vi "Set Control Size.vi"(7 "CtrlRef":refnum<vi>, 9 "Size":cluster{"Width":u32, "Height":u32}, 11 "error in (no error)":errorcluster) -> (15 "error out":errorcluster)   [LabVIEW 2011]
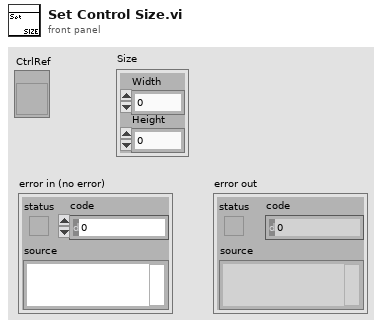
[diagram p1: front panel]
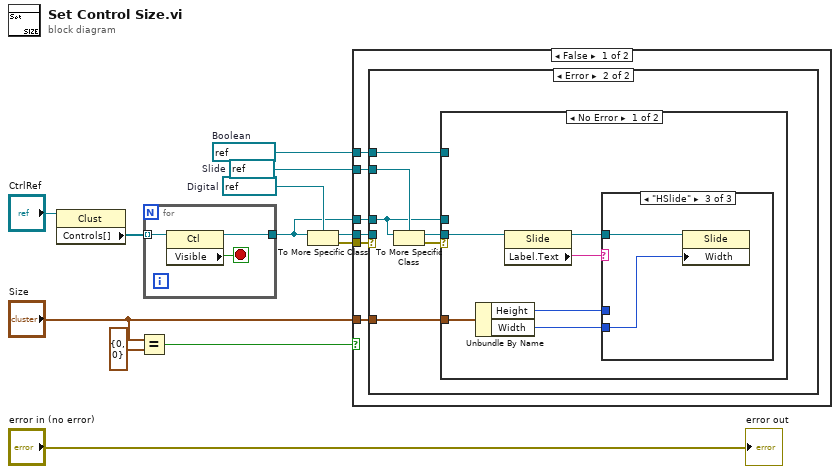
[diagram p0: block diagram]
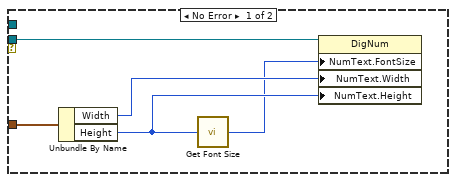
[diagram p2: hidden frame]
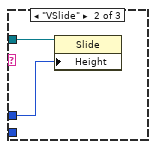
[diagram p4: hidden frame]
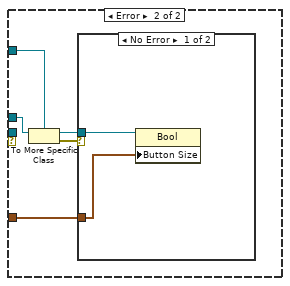
[diagram p5: hidden frame]
diagram:
  w6 = refnum<vi> refnum  # Boolean
  w7 = refnum<vi> refnum  # Slide
  w11 = refnum<vi> refnum  # Digital
  n1 = property class="Clust"(reference="CtrlRef") -> ("Controls[]"=w12:refnum<vi>[])  [unwired: 1 in, 2 out]
  n2 = Equal?(x="Size", y=cluster{"Width":u32, "Height":u32} {"Width"=0, "Height"=0}) -> (x = y?=w1:bool)
  n3 = for {
    tunnel: w12 -> [w15] mode=indexing
    tunnel: [w13] -> w5
    stop <- w14 stop-if-true
    n4 = property class="Ctl"(reference=w15) -> (reference out=w13:refnum<vi>, "Visible"=w14:bool)  [unwired: 1 in, 1 out]
  }
  n5 = To More Specific Class(target class=w11, reference=w5) -> (specific class reference=w8:refnum<vi>, error out=w9:errorcluster)  [unwired: 1 in]
  n6 = case shown="False" w1 {
    tunnel: w9 -> [w21 _]
    tunnel: w8 -> [w20 _]
    tunnel: w7 -> [w19 _]
    tunnel: w6 -> [w18 _]
    tunnel: w5 -> [w17 _]
    tunnel: "Size" -> [w16 _]
    frame False {
      n7 = case shown="Error" w21 {
        tunnel: w20 -> [w26 _]
        tunnel: w19 -> [_ w32]
        tunnel: w18 -> [_ w29]
        tunnel: w16 -> [w25 w28]
        tunnel: w17 -> [_ w27]
        frame No Error {
          n8 = Unbundle By Name(w25) -> ("Width"=w24:u32, "Height"=w23:u32)
          n9 = call "Get Font Size.vi"("Height"=w23) -> ("Font Size"=w22:i32)  [unwired: 14 in]
          n10 = property class="DigNum"(reference=w26, "NumText.FontSize"=w22, "NumText.Width"=w24, "NumText.Height"=w23) -> ()  [unwired: 1 in, 2 out]
        }
        frame Error {
          n11 = To More Specific Class(target class=w32, reference=w27) -> (specific class reference=w31:refnum<vi>, error out=w30:errorcluster)  [unwired: 1 in]
          n12 = case shown="No Error" w30 {
            tunnel: w31 -> [w38 _]
            tunnel: w29 -> [_ w47]
            tunnel: w28 -> [w37 w44]
            tunnel: w27 -> [_ w43]
            frame No Error {
              n13 = Unbundle By Name(w37) -> ("Height"=w36:u32, "Width"=w35:u32)
              n14 = property class="Slide"(reference=w38) -> (reference out=w34:refnum<vi>, "Label.Text"=w33:string)  [unwired: 1 in, 1 out]
              n15 = case shown="\"HSlide\"" w33 {
                tunnel: w36 -> [_ w40 _]
                tunnel: w35 -> [_ _ w42]
                tunnel: w34 -> [_ w39 w41]
                frame "False", Default {
                }
                frame "VSlide" {
                  n16 = property class="Slide"(reference=w39, "Height"=w40) -> ()  [unwired: 1 in, 2 out]
                }
                frame "HSlide" {
                  n17 = property class="Slide"(reference=w41, "Width"=w42) -> ()  [unwired: 1 in, 2 out]
                }
              }
            }
            frame Error {
              n18 = To More Specific Class(target class=w47, reference=w43) -> (specific class reference=w45:refnum<vi>, error out=w46:errorcluster)  [unwired: 1 in]
              n19 = case shown="No Error" w46 {
                tunnel: w45 -> [w49 _]
                tunnel: w44 -> [w48 _]
                frame No Error {
                  n20 = property class="Bool"(reference=w49, "Button Size"=w48) -> ()  [unwired: 1 in, 2 out]
                }
                frame Error {
                }
              }
            }
          }
        }
      }
    }
    frame True {
    }
  }
  "error out" <- "error in (no error)"
